vi "Get Data_old.vi"(8 "error in":errorcluster, 11 "Vaisala Probe in":refnum<class "Vaisala.lvclass">=refnum) -> (0 "error out":errorcluster, 2 "Data Out":refnum<class "Single_Array.lvclass">, 3 "Vaisala Probe out":refnum<class "Vaisala.lvclass">)   [LabVIEW 2014, in "Vaisala.lvclass"]
doc: "Retrieve data from the serial device. The data retrieved should be the standard data for the device, but the structure of that data may differ. This is the reason that an array of data class objects is returned rather than a single value."
uses:
  Vaisala.lvclass
  reusable/Data/Array Data/Single 1-D/Single_Array.lvclass
  Instruments/Nicholas/Session/FPGA Serial Session.lvclass
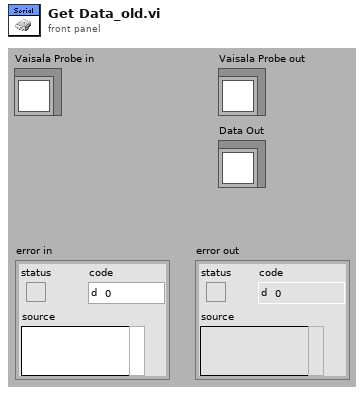
[diagram p1: front panel]
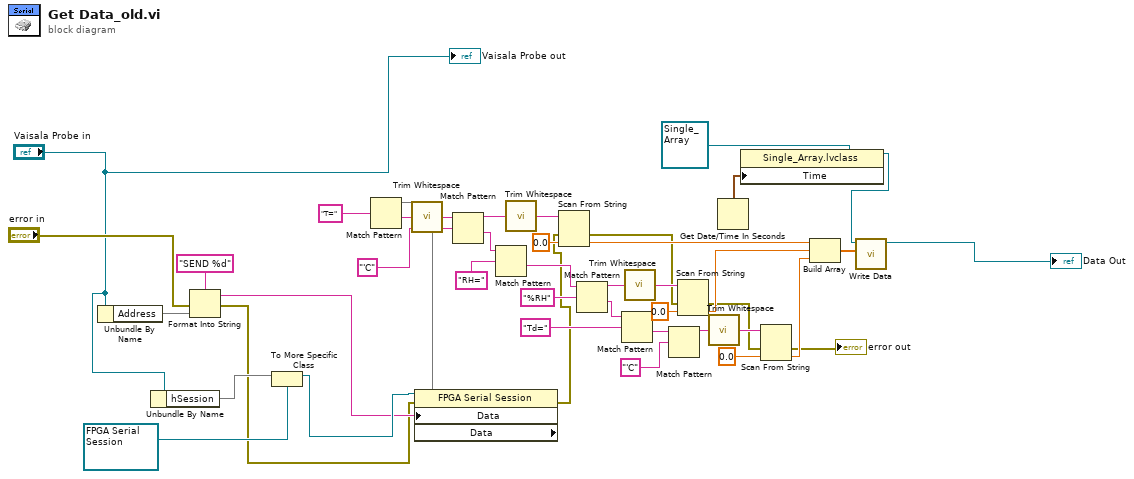
[diagram p0: block diagram]
diagram:
  n1 = Unbundle By Name("Vaisala Probe in") -> ("Address"=w43)
  n2 = Unbundle By Name("Vaisala Probe in") -> ("hSession"=w8)
  n3 = Format Into String(format string="SEND %d", error in="error in", w43) -> (resulting string=w3:string, error out=w2:errorcluster)  [unwired: 1 in]
  n4 = To More Specific Class(target class=refnum<data-value> refnum ("hSession"), reference=w8) -> (specific class reference=w4:refnum<data-value>)  [unwired: 1 in, 1 out]
  n5 = property class="FPGA Serial Session"(reference=w4, error in=w2, "Data"=w3) -> (error out=w1:errorcluster, "Data"=w5)  [unwired: 1 out]
  n6 = Match Pattern(string=w5, regular expression="T=") -> (after substring=w39:string)  [unwired: 1 in, 3 out]
  n7 = call <vilib>:"Trim Whitespace.vi"("string"=w39) -> ("trimmed string"=w38:string)  [unwired: 1 in]
  n8 = Match Pattern(string=w38, regular expression="'C") -> (before substring=w36:string, after substring=w33:string)  [unwired: 1 in, 2 out]
  n9 = Match Pattern(string=w33, regular expression="RH=") -> (after substring=w30:string)  [unwired: 1 in, 3 out]
  n10 = call <vilib>:"Trim Whitespace.vi"("string"=w36) -> ("trimmed string"=w35:string)  [unwired: 1 in]
  n11 = Scan From String(input string=w35, error in=w1, default 1=sgl 0.0 ("output 1")) -> (error out=w15:errorcluster, output 1=w19:sgl)  [unwired: 2 in, 2 out]
  n12 = Match Pattern(string=w30, regular expression="%RH") -> (before substring=w27:string, after substring=w25:string)  [unwired: 1 in, 2 out]
  n13 = Match Pattern(string=w25, regular expression="Td=") -> (after substring=w23:string)  [unwired: 1 in, 3 out]
  n14 = call <vilib>:"Trim Whitespace.vi"("string"=w27) -> ("trimmed string"=w28:string)  [unwired: 1 in]
  n15 = Match Pattern(string=w23, regular expression="'C") -> (before substring=w20:string)  [unwired: 1 in, 3 out]
  n16 = Scan From String(input string=w28, error in=w15, default 1=sgl 0.0 ("output 1")) -> (error out=w14:errorcluster, output 1=w18:sgl)  [unwired: 2 in, 2 out]
  n17 = call <vilib>:"Trim Whitespace.vi"("string"=w20) -> ("trimmed string"=w21:string)  [unwired: 1 in]
  n18 = Get Date/Time In Seconds() -> (seconds since 1Jan1904=w9:timestamp)
  n19 = property class="Single_Array.lvclass"(reference=refnum<class "Single_Array.lvclass"> refnum ("Base Data Class.lvlib:Single_Array.lvclass"), "Time"=w9) -> (reference out=w10:refnum<class "Single_Array.lvclass">)  [unwired: 1 in, 1 out]
  n20 = Scan From String(input string=w21, error in=w14, default 1=sgl 0.0 ("output 1")) -> (error out=→"error out":errorcluster, output 1=w17:sgl)  [unwired: 2 in, 2 out]
  n21 = Build Array(w19, w18, w17) -> (w16:sgl[])
  n22 = call "Write Data.vi"("Data"=w16, "Single_Array in"=w10) -> ("Single_Array out"=→"Data Out":refnum<class "Single_Array.lvclass">)  [unwired: 8 in, 1 out]
  "Vaisala Probe out" <- "Vaisala Probe in"
